vi "Main.vi"() -> ()   [LabVIEW 2019]
panel:
  out "Time has elapsed?":bool
  in  "Start":bool
  out "Elapsed time (s)":dbl=5.0 format="%#_2g"
  in  "Time target (s)":dbl=5.0
  in  "Stop":bool
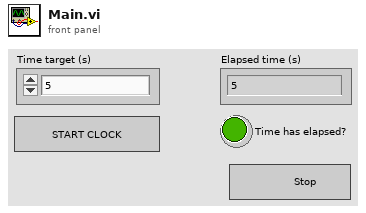
[diagram p1: front panel]
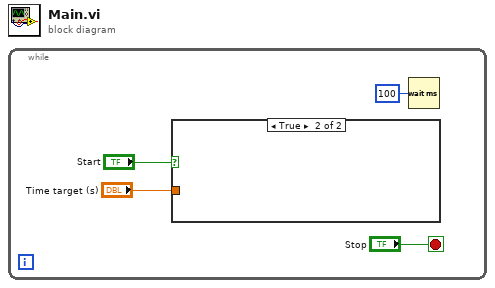
[diagram p0: block diagram]
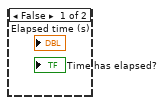
[diagram p2: hidden frame]
diagram:
  n1 = while {
    stop <- "Stop" stop-if-true
    n2 = case shown="True" "Start" {
      tunnel: "Time target (s)" -> [_ _]
      frame False {
      }
      frame True {
      }
    }
    n3 = Wait (ms)(milliseconds to wait=u32 100) -> ()  [unwired: 1 out]
  }
